vi "ZVL Network Analyser - data acquisition fstart to fend .vi"(8 "error in (no error)":errorcluster) -> (0 "error out":errorcluster, 1 "N segments":i32, 2 "Data array {Freq}{Real}{Imag}":string[](array[string]))   [LabVIEW 2019]
doc: "Nicolas Weiss - EPFL - IPHYS 2019\n----\nThis VI performs a data acquisition with the ZVL network analyzer on the fequency range defined by the user [startf, stopf] (set through golbal variables).\nDue to device limitation, the full frequency range is divided into smaller frenquency segments [newStarting, newEnding]."
uses:
  bf107b11-901b-45e0-a3a2-c4b682ef9b8c.vi
  _Global variables 1.vi
panel:
  in  "String":string
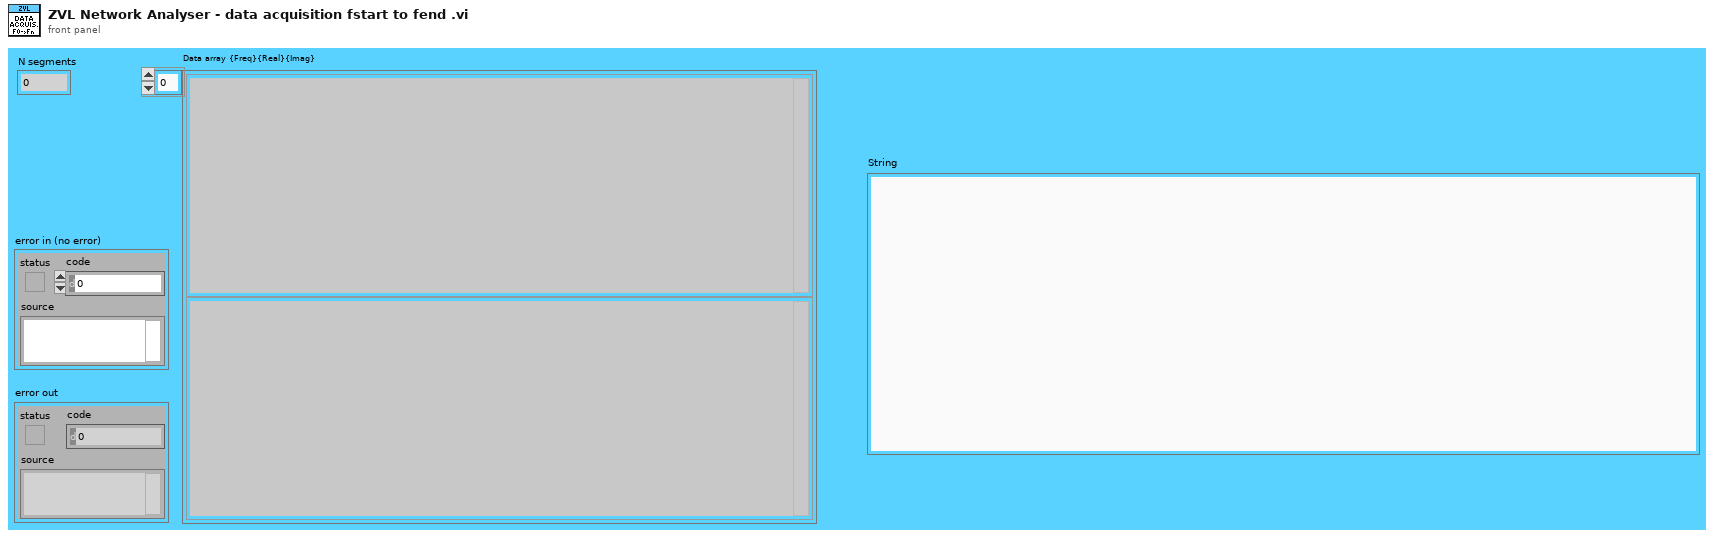
[diagram p1: front panel]
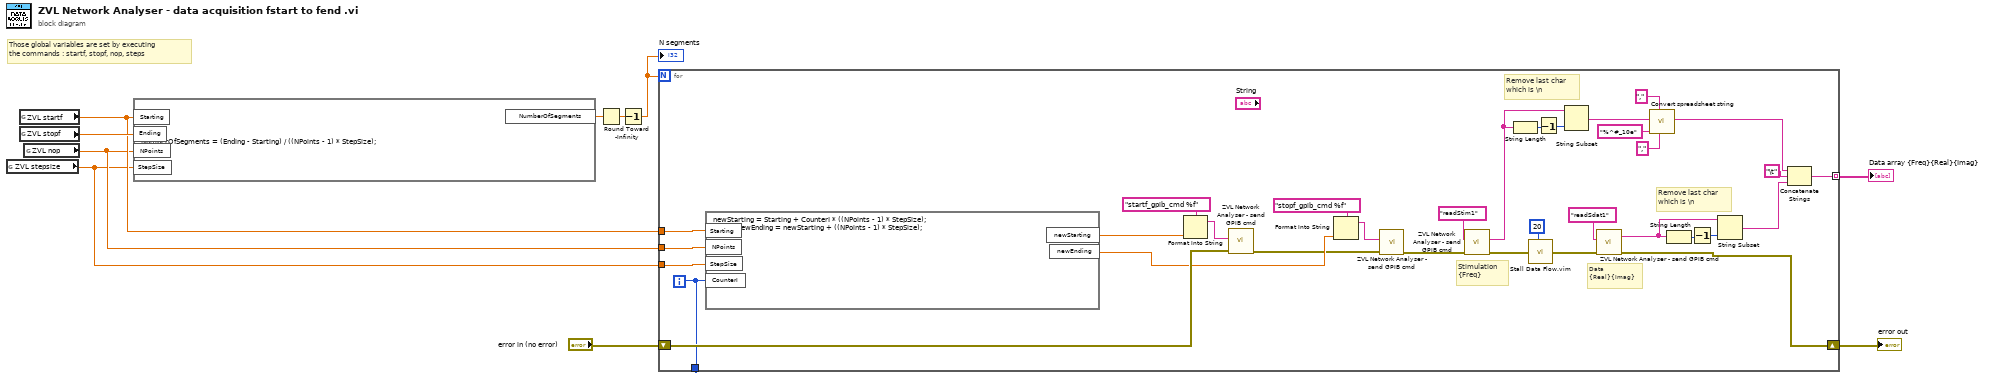
[diagram p0: block diagram]
diagram:
  # "Those global variables are set by executing \nthe commands : startf, stopf, nop, steps"
  n1 = global read "_Global variables 1.vi" "ZVL stepsize"() -> (w7:dbl)
  n2 = global read "_Global variables 1.vi" "ZVL startf"() -> (w9:dbl)
  n3 = global read "_Global variables 1.vi" "ZVL stopf"() -> (w10:dbl)
  n4 = global read "_Global variables 1.vi" "ZVL nop"() -> (w8:dbl)
  n5 = formula code="NumberOfSegments = (Ending - Starting) / ((NPoints - 1) * StepSize);"("Starting"=w9, "Ending"=w10, "NPoints"=w8, "StepSize"=w7) -> ("NumberOfSegments"=w6:dbl)
  n6 = Round Toward -Infinity(1:w6) -> (0:w5:dbl)
  n7 = Decrement(x=w5) -> (x-1=w1:dbl)
  "N segments" <- w1
  n8 = for {
    N: w1 -> [_]
    tunnel: w9 -> [w43]
    tunnel: w8 -> [w42]
    tunnel: w7 -> [w41]
    tunnel: [w29] -> w2 mode=indexing
    shift-right: [w21] -> w3
    shift-left: "error in (no error)" -> [w40]
    tunnel: [w16] -> _
    i -> [w16]
    # "Stimulation\n{Freq}"
    # "Data\n{Real}{Imag}"
    # "Remove last char\nwhich is \\n"
    # "Remove last char\nwhich is \\n"
    n9 = formula code="newStarting = Starting + CounterI * ((NPoints - 1) * StepSize);\n            newEnding = newStarting + ((NPoints - 1) * StepSize);"("Starting"=w43, "NPoints"=w42, "StepSize"=w41, "CounterI"=w16) -> ("newStarting"=w38:dbl, "newEnding"=w34:dbl)
    n10 = Format Into String(format string="startf_gpib_cmd %f", w38) -> (resulting string=w37:string)  [unwired: 2 in, 1 out]
    n11 = call "ZVL Network Analyser - send GPIB cmd.vi"("error in (no error)"=w40, "Cmd string"=w37) -> ("error out"=w33:errorcluster)  [unwired: 8 in, 1 out]
    n12 = Format Into String(format string="stopf_gpib_cmd %f", w34) -> (resulting string=w36:string)  [unwired: 2 in, 1 out]
    n13 = call "ZVL Network Analyser - send GPIB cmd.vi"("error in (no error)"=w33, "Cmd string"=w36) -> ("error out"=w25:errorcluster)  [unwired: 8 in, 1 out]
    n14 = call "ZVL Network Analyser - send GPIB cmd.vi"("error in (no error)"=w25, "Cmd string"="readStim1" ("format string")) -> ("error out"=w24:errorcluster, "Response"=w28:string)  [unwired: 8 in]
    n15 = String Length(string=w28) -> (length=w27:i32)
    n16 = call "Stall Data Flow.vim"("value in"=w24, "milliseconds to wait"=u32 20) -> ("value out"=w23:errorcluster)  [unwired: 1 out]
    n17 = Decrement(x=w27) -> (x-1=w26:i32)
    n18 = String Subset(string=w28, length (rest)=w26) -> (substring=w15:string)  [unwired: 1 in]
    n19 = call "ZVL Network Analyser - send GPIB cmd.vi"("error in (no error)"=w23, "Cmd string"="readSdat1" ("format string")) -> ("error out"=w21:errorcluster, "Response"=w18:string)  [unwired: 8 in]
    n20 = call "Convert spreadsheet string.vi"("Delimiter [output]"=",", "Delimiter [input]"=",", "Format [output]"="%^#_10e", "List of numbers [input]"=w15) -> ("List of numbers [output]"=w14:string)  [unwired: 6 in, 1 out]
    n21 = String Length(string=w18) -> (length=w19:i32)
    n22 = Decrement(x=w19) -> (x-1=w20:i32)
    n23 = String Subset(string=w18, length (rest)=w20) -> (substring=w17:string)  [unwired: 1 in]
    n24 = Concatenate Strings(w14, "\t" ("string"), w17) -> (w29:string)
  }
  "error out" <- w3
  "Data array {Freq}{Real}{Imag}" <- w2
